vi "VI Tree.vi"   [LabVIEW 2010, in "Yudian AI508.lvlib"]
doc: "This is the instrument driver for the <INSTRUMENT NAME>. The VI Tree displays all the user-callable VIs of the instrument driver in an organized table."
uses:
  <instrlib>/Yudian AI508/Yudian AI508.lvlib
panel:
  # "(c) 2014 Microscale Transport Lab.  ALL RIGHTS RESERVED."
  # "SEE DIAGRAM\nFOR VI TREE."
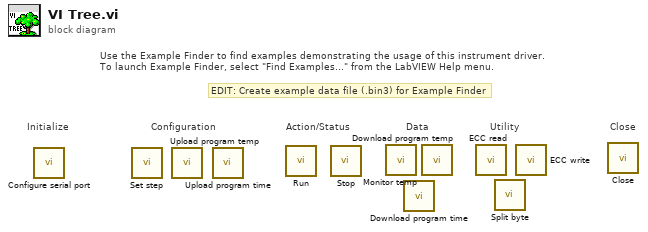
[diagram p0: block diagram]
diagram:
  # "EDIT: Create example data file (.bin3) for Example Finder"
  # "Use the Example Finder to find examples demonstrating the usage of this instrument driver.\nTo launch Example Finder, select \"Find Examples...\" from the LabVIEW Help menu."
  # "Configuration"
  # "Utility"
  # "Data"
  # "Action/Status"
  # "Close"
  # "Initialize"
  n1 = call <instrlib>:"Configure serial port.vi"() -> ()  [unwired: 10 in, 2 out]
  n2 = call <instrlib>:"Set step.vi"() -> ()  [unwired: 10 in, 2 out]
  n3 = call <instrlib>:"Upload program temp.vi"() -> ()  [unwired: 10 in, 2 out]
  n4 = call <instrlib>:"Upload program time.vi"() -> ()  [unwired: 10 in, 2 out]
  n5 = call <instrlib>:"Run.vi"() -> ()  [unwired: 10 in, 2 out]
  n6 = call <instrlib>:"Stop.vi"() -> ()  [unwired: 10 in, 2 out]
  n7 = call <instrlib>:"Monitor temp.vi"() -> ()  [unwired: 9 in, 3 out]
  n8 = call <instrlib>:"Download program time.vi"() -> ()  [unwired: 9 in, 3 out]
  n9 = call <instrlib>:"Download program temp.vi"() -> ()  [unwired: 9 in, 3 out]
  n10 = call <instrlib>:"ECC read.vi"() -> ()  [unwired: 11 in, 1 out]
  n11 = call <instrlib>:"Split byte.vi"() -> ()  [unwired: 11 in, 1 out]
  n12 = call <instrlib>:"ECC write.vi"() -> ()  [unwired: 11 in, 1 out]
  n13 = call <instrlib>:"Close.vi"() -> ()  [unwired: 11 in, 1 out]
